vi "TRIG_CHAN_AUX_DUR.vi"(0 "VISA IN":refnum<visa-resource-name>, 1 "Aux":i32, 2 "Duration":dbl, 5 "error in":errorcluster, 7 "Channel":i32) -> (14 "VISA Out":refnum<visa-resource-name>, 19 "error out":errorcluster)   [LabVIEW 2018, in "PNA-X.lvlib"]
doc: "TRIGger:CHANnel<ch>:AUX<n>:DURation <num> \n(Read-Write) Specifies the width of the output pulse, which is the time that the Aux trigger output \nwill be asserted. \nParameters \n<ch> Any existing channel number. If unspecified, value is set to 1. \n<n> Rear panel connector used to send or receive signals. \nPNA-X - choose from 1 (AUX TRIG 1) or 2 (AUX TRIG 2) \nAll other models: choose 1. (BNC Trig I/O \nIf unspecified, value is set to 1. \n<num> Duration value in seconds. Choose a value between 1us (1E-6) and 1 \nExamples TRIG:CHAN:AUX:DUR .1 \ntrigger:channel2:aux2:duration .01 \nQuery Syntax TRIGger:CHANnel<ch>:AUX<n>:DURation? \nReturn Type Numeric \nDefault 1E-6"
uses:
  PNA-X.lvlib
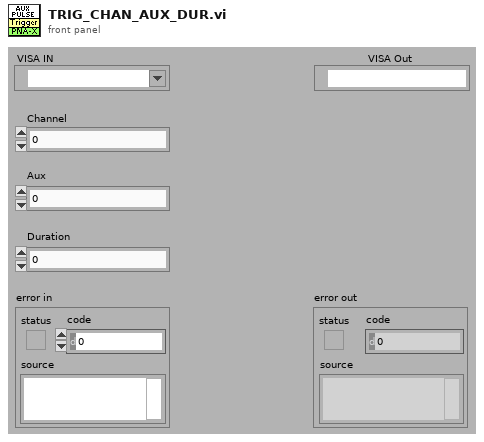
[diagram p1: front panel]
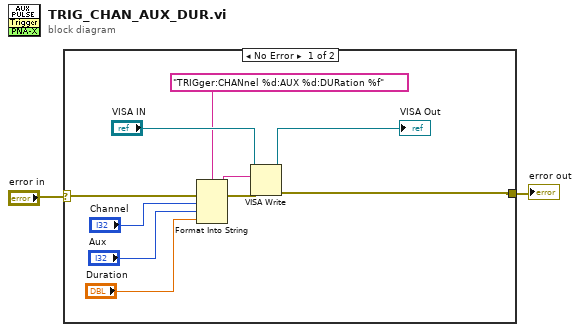
[diagram p0: block diagram]
diagram:
  n1 = case shown="No Error" "error in" {
    selector: "error in" -> [w12 w13]
    tunnel: [w7 w13] -> w1
    frame No Error {
      n2 = Format Into String(format string="TRIGger:CHANnel %d:AUX %d:DURation %f" ("Cmdline"), error in=w12, "Channel", "Aux", "Duration") -> (resulting string=w10:string, error out=w11:errorcluster)  [unwired: 1 in]
      n3 = VISA Write(VISA resource name="VISA IN", write buffer=w10, error in (no error)=w11) -> (VISA resource name out=→"VISA Out":refnum<visa-resource-name>, error out=w7:errorcluster)  [unwired: 1 out]
    }
    frame Error {
    }
  }
  "error out" <- w1
